vi "Ring-shaped Horizontal Lines.vi"(8 "error in (no error)":errorcluster, 9 "Separation (angle)":dbl=5.0, 10 "Vert. Line Length":i32=300, 11 "Revolution (steps)":i32=3200) -> (0 "error out":errorcluster)   [LabVIEW 2017]
doc: "To draw horizontal lines around the round object."
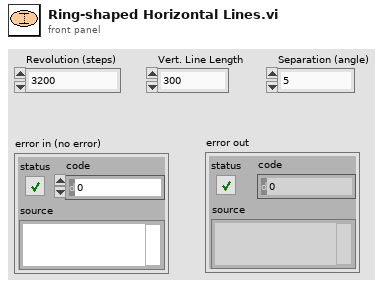
[diagram p1: front panel]
types:
  T1 = enum16{"Full", "Half", "Quarter", "Eighth", "Sixteenth"}
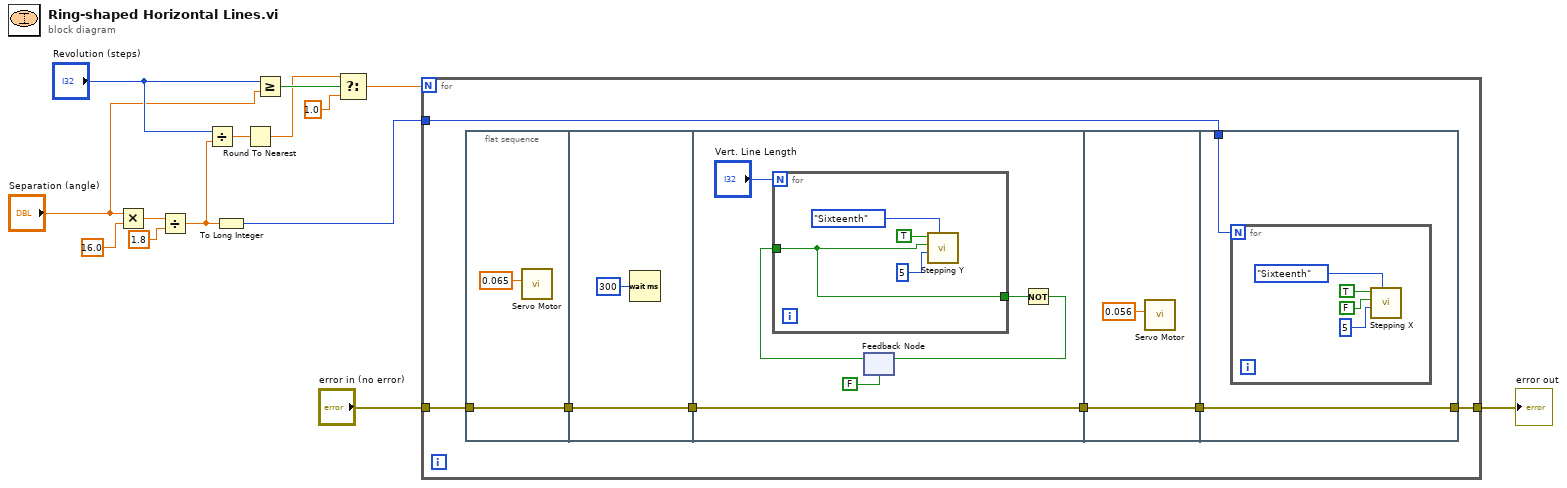
[diagram p0: block diagram]
diagram:
  n1 = Multiply(x="Separation (angle)", y=16.0) -> (x*y=w10:dbl)
  n2 = Divide(x=w10, y=1.8) -> (x/y=w7:dbl)
  n3 = Divide(x="Revolution (steps)", y=w7) -> (x/y=w14:dbl)
  n4 = To Long Integer(number=w7) -> (32bit integer=w8:i32)
  n5 = Round To Nearest(number=w14) -> (nearest integer value=w2:dbl)
  n6 = Greater Or Equal?(x="Revolution (steps)", y="Separation (angle)") -> (x >= y?=w4:bool)
  n7 = Select(t=w2, s=w4, f=1.0) -> (s? t:f=w6:dbl)
  n8 = for {
    N: w6 -> [_]
    tunnel: w8 -> [w21]
    tunnel: "error in (no error)" -> [w19]
    tunnel: [w15] -> w12
    n9 = flat-sequence {
      tunnel: [w22] -> w20
      tunnel: w19 -> [w22]
      tunnel: w20 -> [w24]
      tunnel: [w24] -> w18
      tunnel: w18 -> [w26]
      tunnel: [w26] -> w16
      tunnel: [w36] -> w17
      tunnel: w16 -> [w36]
      tunnel: w21 -> [w39]
      tunnel: w17 -> [w38]
      tunnel: [w38] -> w15
      frame #0 {
        n10 = call "Servo Motor.vi"("Duty Cycle"=0.065) -> ()  [unwired: 10 in, 1 out]
      }
      frame #1 {
        n11 = Wait (ms)(milliseconds to wait=u32 300) -> ()  [unwired: 1 out]
      }
      frame #2 {
        n12 = feedback #1(FALSE) -> (w29:bool)
        n13 = for {
          N: "Vert. Line Length" -> [_]
          tunnel: w29 -> [w32]
          tunnel: [w32] -> w28
          n14 = call "Stepping Y.vi"("Microstep size"=T1."Sixteenth", "Speed"=u32 5, "Direction"=w32, "Enable"=TRUE) -> ()  [unwired: 7 in, 1 out]
        }
        n15 = Not(x=w28) -> (.not. x?=w27:bool)
        n16 = feedback-in #1(w27) -> ()
      }
      frame #3 {
        n17 = call "Servo Motor.vi"("Duty Cycle"=0.056) -> ()  [unwired: 10 in, 1 out]
      }
      frame #4 {
        n18 = for {
          N: w39 -> [_]
          n19 = call "Stepping X.vi"("Microstep size"=T1."Sixteenth", "Speed"=u32 5, "Direction"=FALSE, "Enable"=TRUE) -> ()  [unwired: 7 in, 1 out]
        }
      }
    }
  }
  "error out" <- w12
